vi "References.vi"(8 "error in":errorcluster, 10 "variant":variant, 11 "Reference AE Control":T2=enum."Set Profile") -> (0 "error out":errorcluster, 3 "Cluster out":T1)   [LabVIEW 2013, in "main.lvlib"]
uses:
  main.lvlib
  Controls/Reference AE Control.ctl
  Controls/Reference Cluster.ctl
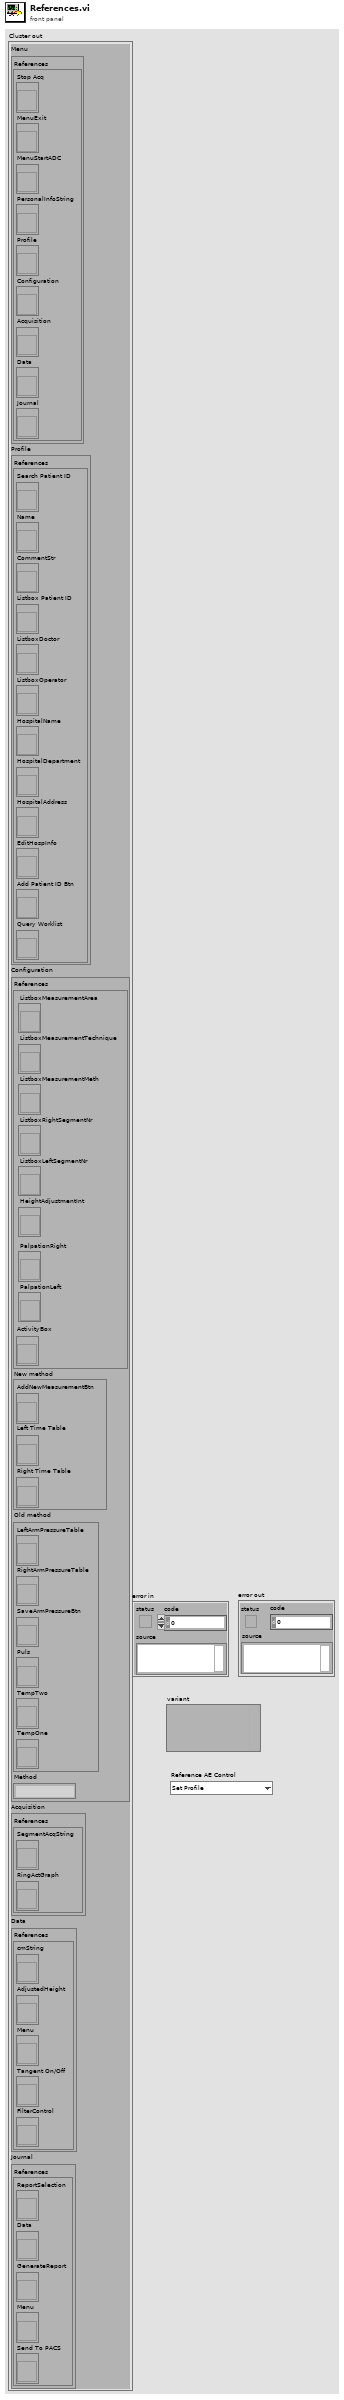
[diagram p1: front panel]
types:
  T1 = typedef "main.lvlib/Reference Cluster.ctl" = cluster{"Menu":cluster{"References":cluster{"Stop Acq":refnum<vi>, "MenuExit":refnum<vi>, "MenuStartADC":refnum<vi>, "PersonalInfoString":refnum<vi>, "Profile":refnum<vi>, "Configuration":refnum<vi>, "Acquisition":refnum<vi>, "Data":refnum<vi>, "Journal":refnum<vi>}}, "Profile":cluster{"References":cluster{"Search Patient ID":refnum<vi>, "Name":refnum<vi>, "CommentStr":refnum<vi>, "Listbox Patient ID":refnum<vi>, "ListboxDoctor":refnum<vi>, "ListboxOperator":refnum<vi>, "HospitalName":refnum<vi>, "HospitalDepartment":refnum<vi>, "HospitalAddress":refnum<vi>, "EditHospInfo":refnum<vi>, "Add Patient ID Btn":refnum<vi>, "Query Worklist":refnum<vi>}}, "Configuration":cluster{"References":cluster{"ListboxMeasurementArea":refnum<vi>, "ListboxMeasurementTechnique":refnum<vi>, "ListboxMeasurementMeth":refnum<vi>, "ListboxRightSegmentNr":refnum<vi>, "ListboxLeftSegmentNr":refnum<vi>, "HeightAdjustmentInt":refnum<vi>, "PalpationRight":refnum<vi>, "PalpationLeft":refnum<vi>, "ActivityBox":refnum<vi>}, "New method":cluster{"AddNewMeasurementBtn":refnum<vi>, "Left Time Table":refnum<vi>, "Right Time Table":refnum<vi>}, "Old method":cluster{"LeftArmPressureTable":refnum<vi>, "RightArmPressureTable":refnum<vi>, "SaveArmPressureBtn":refnum<vi>, "Puls":refnum<vi>, "TempTwo":refnum<vi>, "TempOne":refnum<vi>}, "Method":string}, "Acquisition":cluster{"References":cluster{"SegmentAcqString":refnum<vi>, "RingActGraph":refnum<vi>}}, "Data":cluster{"References":cluster{"cmString":refnum<vi>, "AdjustedHeight":refnum<vi>, "Menu":refnum<vi>, "Tangent On/Off":refnum<vi>, "FilterControl":refnum<vi>}}, "Journal":cluster{"References":cluster{"ReportSelection":refnum<vi>, "Data":refnum<vi>, "GenerateReport":refnum<vi>, "Menu":refnum<vi>, "Send To PACS":refnum<vi>}}}
  T2 = typedef "main.lvlib/Reference AE Control.ctl" = enum16{"Initialize", "Set Menu", "Set Profile", "Set Configuration", "Set Configuration_old", "Set Configuration_new", "Set Configuration Method", "Set Acquisition", "Set Data", "Set Journal", "Get"}
  T3 = cluster{"Stop Acq":refnum<vi>, "MenuExit":refnum<vi>, "MenuStartADC":refnum<vi>, "PersonalInfoString":refnum<vi>, "Profile":refnum<vi>, "Configuration":refnum<vi>, "Acquisition":refnum<vi>, "Data":refnum<vi>, "Journal":refnum<vi>}
  T4 = cluster{"Search Patient ID":refnum<vi>, "Name":refnum<vi>, "CommentStr":refnum<vi>, "Listbox Patient ID":refnum<vi>, "ListboxDoctor":refnum<vi>, "ListboxOperator":refnum<vi>, "HospitalName":refnum<vi>, "HospitalDepartment":refnum<vi>, "HospitalAddress":refnum<vi>, "EditHospInfo":refnum<vi>, "Add Patient ID Btn":refnum<vi>, "Query Worklist":refnum<vi>}
  T5 = cluster{"ListboxMeasurementArea":refnum<vi>, "ListboxMeasurementTechnique":refnum<vi>, "ListboxMeasurementMeth":refnum<vi>, "ListboxRightSegmentNr":refnum<vi>, "ListboxLeftSegmentNr":refnum<vi>, "HeightAdjustmentInt":refnum<vi>, "PalpationRight":refnum<vi>, "PalpationLeft":refnum<vi>, "ActivityBox":refnum<vi>}
  T6 = cluster{"LeftArmPressureTable":refnum<vi>, "RightArmPressureTable":refnum<vi>, "SaveArmPressureBtn":refnum<vi>, "Puls":refnum<vi>, "TempTwo":refnum<vi>, "TempOne":refnum<vi>}
  T7 = cluster{"AddNewMeasurementBtn":refnum<vi>, "Left Time Table":refnum<vi>, "Right Time Table":refnum<vi>}
  T8 = cluster{"SegmentAcqString":refnum<vi>, "RingActGraph":refnum<vi>}
  T9 = cluster{"cmString":refnum<vi>, "AdjustedHeight":refnum<vi>, "Menu":refnum<vi>, "Tangent On/Off":refnum<vi>, "FilterControl":refnum<vi>}
  T10 = cluster{"ReportSelection":refnum<vi>, "Data":refnum<vi>, "GenerateReport":refnum<vi>, "Menu":refnum<vi>, "Send To PACS":refnum<vi>}
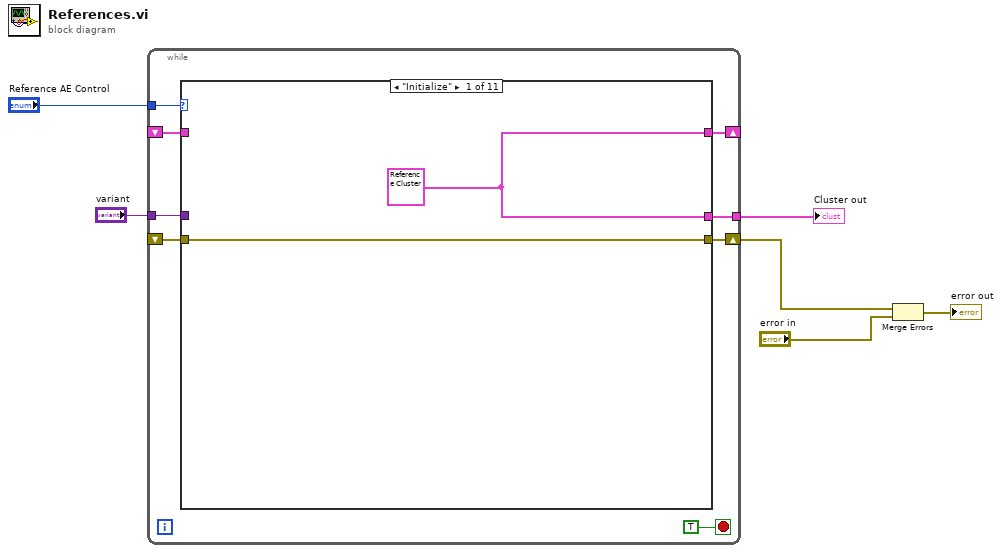
[diagram p0: block diagram]
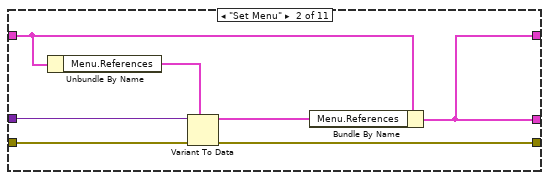
[diagram p2: hidden frame]
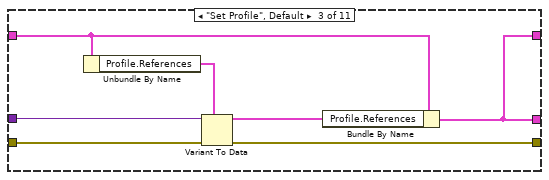
[diagram p3: hidden frame]
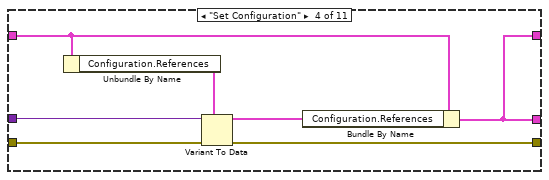
[diagram p4: hidden frame]
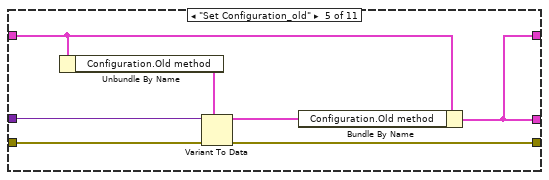
[diagram p5: hidden frame]
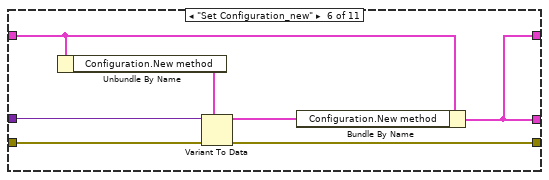
[diagram p6: hidden frame]
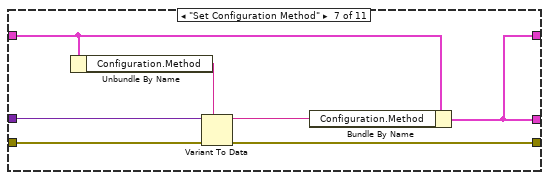
[diagram p7: hidden frame]
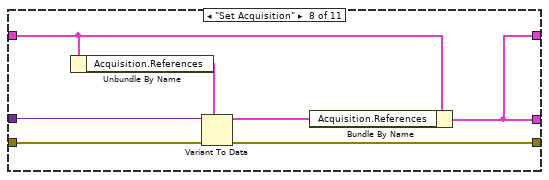
[diagram p8: hidden frame]
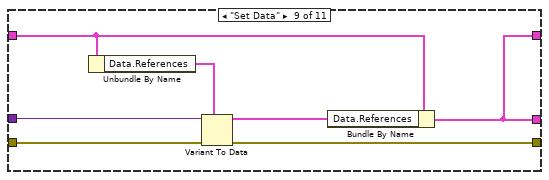
[diagram p9: hidden frame]
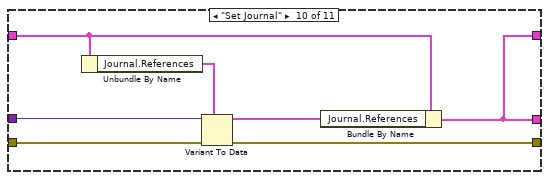
[diagram p10: hidden frame]
diagram:
  n1 = while {
    tunnel: "Reference AE Control" -> [w14]
    shift-right: [w11] -> _
    shift-left: _ -> [w13]
    tunnel: "variant" -> [w12]
    tunnel: [w10] -> w4
    shift-right: [w7] -> w2
    shift-left: _ -> [w8]
    stop <- TRUE stop-if-true
    n2 = case shown="\"Initialize\"" w14 {
      tunnel: w13 -> [_ w20 w28 w35 w42 w49 w56 w63 w70 w77 w81]
      tunnel: w12 -> [_ w22 w30 w37 w44 w51 w58 w65 w72 w79 _]
      tunnel: [w16 w21 w26 w33 w40 w47 w54 w61 w68 w75 w81] -> w11
      tunnel: [w16 w21 w26 w33 w40 w47 w54 w61 w68 w75 w81] -> w10
      tunnel: w8 -> [w15 w18 w25 w32 w39 w46 w53 w60 w67 w74 w80]
      tunnel: [w15 w17 w24 w31 w38 w45 w52 w59 w66 w73 w80] -> w7
      frame "Initialize" {
        w16 = T1 {"Menu"={"References"={"Stop Acq"=refnum, "MenuExit"=refnum, "MenuStartADC"=refnum, "PersonalInfoString"=refnum, "Profile"=refnum, "Configuration"=refnum, "Acquisition"=refnum, "Data"=refnum, "Journal"=refnum}}, "Profile"={"References"={"Search Patient ID"=refnum, "Name"=refnum, "CommentStr"=refnum, "Listbox Patient ID"=refnum, "ListboxDoctor"=refnum, "ListboxOperator"=refnum, "HospitalName"=refnum, "HospitalDepartment"=refnum, "HospitalAddress"=refnum, "EditHospInfo"=refnum, "Add Patient ID Btn"=refnum, "Query Worklist"=refnum}}, "Configuration"={"References"={"ListboxMeasurementArea"=refnum, "ListboxMeasurementTechnique"=refnum, "ListboxMeasurementMeth"=refnum, "ListboxRightSegmentNr"=refnum, "ListboxLeftSegmentNr"=refnum, "HeightAdjustmentInt"=refnum, "PalpationRight"=refnum, "PalpationLeft"=refnum, "ActivityBox"=refnum}, "New method"={"AddNewMeasurementBtn"=refnum, "Left Time Table"=refnum, "Right Time Table"=refnum}, "Old method"={"LeftArmPressureTable"=refnum, "RightArmPressureTable"=refnum, "SaveArmPressureBtn"=refnum, "Puls"=refnum, "TempTwo"=refnum, "TempOne"=refnum}, "Method"=""}, "Acquisition"={"References"={"SegmentAcqString"=refnum, "RingActGraph"=refnum}}, "Data"={"References"={"cmString"=refnum, "AdjustedHeight"=refnum, "Menu"=refnum, "Tangent On/Off"=refnum, "FilterControl"=refnum}}, "Journal"={"References"={"ReportSelection"=refnum, "Data"=refnum, "GenerateReport"=refnum, "Menu"=refnum, "Send To PACS"=refnum}}}
      }
      frame "Set Menu" {
        n3 = Unbundle By Name(w20) -> ("Menu.References"=w23:T3)
        n4 = Variant To Data(error in=w18, type=w23, Variant=w22) -> (data=w19:T3, error out=w17:errorcluster)
        n5 = Bundle By Name(cluster=w20, "Menu.References"=w19) -> (w21:T1)
      }
      frame "Set Profile", Default {
        n6 = Unbundle By Name(w28) -> ("Profile.References"=w29:T4)
        n7 = Variant To Data(error in=w25, type=w29, Variant=w30) -> (data=w27:T4, error out=w24:errorcluster)
        n8 = Bundle By Name(cluster=w28, "Profile.References"=w27) -> (w26:T1)
      }
      frame "Set Configuration" {
        n9 = Unbundle By Name(w35) -> ("Configuration.References"=w36:T5)
        n10 = Variant To Data(error in=w32, type=w36, Variant=w37) -> (data=w34:T5, error out=w31:errorcluster)
        n11 = Bundle By Name(cluster=w35, "Configuration.References"=w34) -> (w33:T1)
      }
      frame "Set Configuration_old" {
        n12 = Unbundle By Name(w42) -> ("Configuration.Old method"=w43:T6)
        n13 = Variant To Data(error in=w39, type=w43, Variant=w44) -> (data=w41:T6, error out=w38:errorcluster)
        n14 = Bundle By Name(cluster=w42, "Configuration.Old method"=w41) -> (w40:T1)
      }
      frame "Set Configuration_new" {
        n15 = Unbundle By Name(w49) -> ("Configuration.New method"=w50:T7)
        n16 = Variant To Data(error in=w46, type=w50, Variant=w51) -> (data=w48:T7, error out=w45:errorcluster)
        n17 = Bundle By Name(cluster=w49, "Configuration.New method"=w48) -> (w47:T1)
      }
      frame "Set Configuration Method" {
        n18 = Unbundle By Name(w56) -> ("Configuration.Method"=w57:string)
        n19 = Variant To Data(error in=w53, type=w57, Variant=w58) -> (data=w55:string, error out=w52:errorcluster)
        n20 = Bundle By Name(cluster=w56, "Configuration.Method"=w55) -> (w54:T1)
      }
      frame "Set Acquisition" {
        n21 = Unbundle By Name(w63) -> ("Acquisition.References"=w64:T8)
        n22 = Variant To Data(error in=w60, type=w64, Variant=w65) -> (data=w62:T8, error out=w59:errorcluster)
        n23 = Bundle By Name(cluster=w63, "Acquisition.References"=w62) -> (w61:T1)
      }
      frame "Set Data" {
        n24 = Unbundle By Name(w70) -> ("Data.References"=w71:T9)
        n25 = Variant To Data(error in=w67, type=w71, Variant=w72) -> (data=w69:T9, error out=w66:errorcluster)
        n26 = Bundle By Name(cluster=w70, "Data.References"=w69) -> (w68:T1)
      }
      frame "Set Journal" {
        n27 = Unbundle By Name(w77) -> ("Journal.References"=w78:T10)
        n28 = Variant To Data(error in=w74, type=w78, Variant=w79) -> (data=w76:T10, error out=w73:errorcluster)
        n29 = Bundle By Name(cluster=w77, "Journal.References"=w76) -> (w75:T1)
      }
      frame "Get" {
      }
    }
  }
  "Cluster out" <- w4
  n30 = Merge Errors(w2, "error in") -> (→"error out":errorcluster)
